vi "test.vi"() -> ()   [LabVIEW 2020]
panel:
  out "Array":string[](array[string])
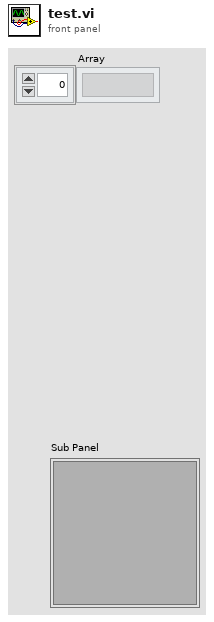
[diagram p1: front panel]
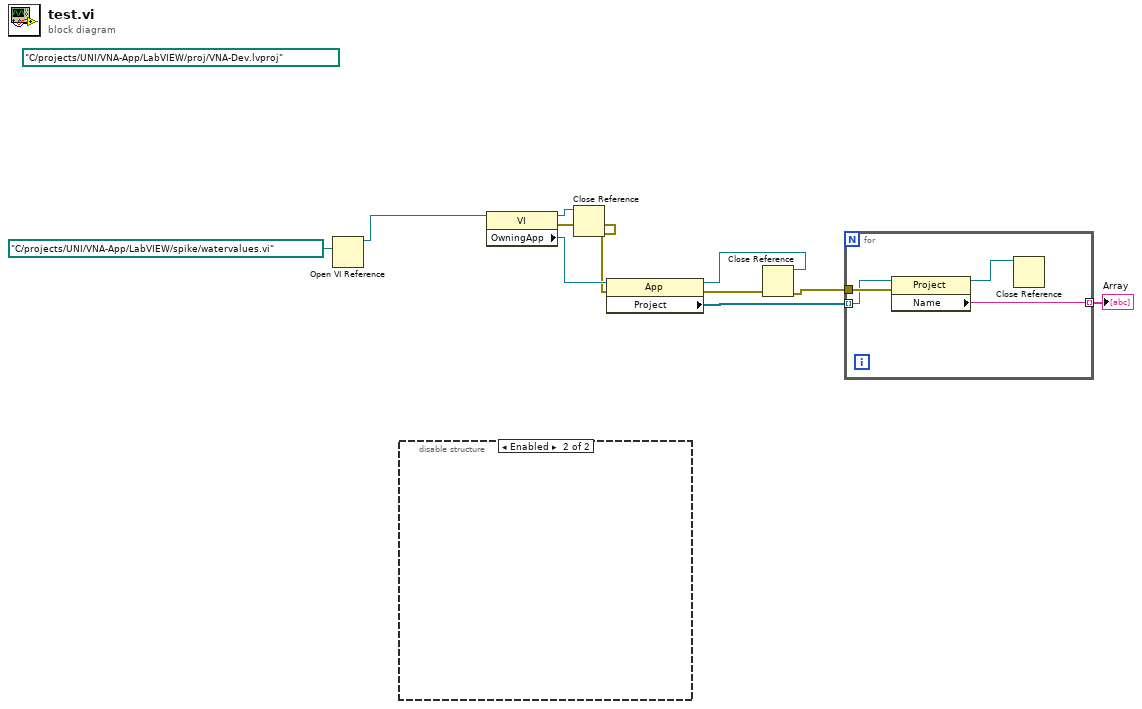
[diagram p0: block diagram]
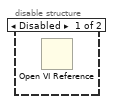
[diagram p2: hidden frame]
diagram:
  (unwired) path "C:/projects/UNI/VNA-App/LabVIEW/proj/VNA-Dev.lvproj" ("Path")
  n1 = Open VI Reference(vi path=path "C:/projects/UNI/VNA-App/LabVIEW/spike/watervalues.vi") -> (vi reference=w10:refnum<vi>)  [unwired: 5 in, 1 out]
  n2 = disable-structure shown="Enabled" {
    frame Disabled {
      n3 = Open VI Reference() -> ()  [unwired: 6 in, 2 out]
    }
    frame Enabled {
    }
  }
  n4 = property class="VI"(reference=w10) -> (reference out=w7:refnum<vi>, error out=w6:errorcluster, "OwningApp"=w9:refnum<vi>)  [unwired: 1 in]
  n5 = Close Reference(reference=w7, error in (no error)=w6) -> (error out=w5:errorcluster)
  n6 = property class="App"(reference=w9, error in=w5) -> (reference out=w3:refnum<vi>, error out=w4:errorcluster, "Project"=w8:refnum<vi>[])
  n7 = Close Reference(reference=w3, error in (no error)=w4) -> (error out=w2:errorcluster)
  n8 = for {
    tunnel: w8 -> [w14] mode=indexing
    tunnel: w2 -> [w15]
    tunnel: [w13] -> w1 mode=indexing
    n9 = property class="Project"(reference=w14, error in=w15) -> (reference out=w12:refnum<vi>, "Name"=w13:string)  [unwired: 1 out]
    n10 = Close Reference(reference=w12) -> ()  [unwired: 1 in, 1 out]
  }
  "Array" <- w1
